vi "Check is Supported.vi"(10 "desired font(Application)":T2(ring), 11 "[user-specified font]":T1) -> (3 "is_supported":bool)   [LabVIEW 2021, in "Picture Pixel Fonts.lvlib"]
uses:
  <vilib>/LabVIEW Icon API/Pixel Fonts/Picture Pixel Fonts.lvlib
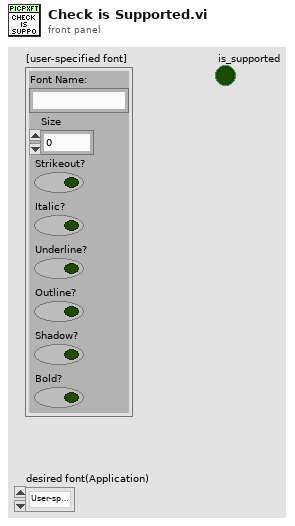
[diagram p1: front panel]
types:
  T1 = cluster{"Font Name:":string, "Size":i16, "Strikeout?":bool, "Italic?":bool, "Underline?":bool, "Outline?":bool, "Shadow?":bool, "Bold?":bool}
  T2 = enum16{"User-specified Font", "Application Font", "System Font", "Dialog Font"}
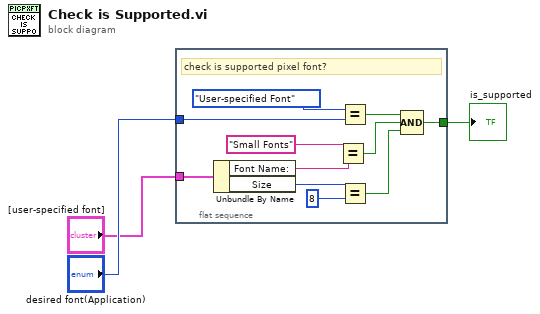
[diagram p0: block diagram]
diagram:
  n1 = flat-sequence {
    tunnel: "[user-specified font]" -> [w14]
    tunnel: "desired font(Application)" -> [w12]
    tunnel: [w4] -> w3
    frame #0 {
      # "check is supported pixel font?"
      n2 = Unbundle By Name(w14) -> ("Font Name:"=w11:string, "Size"=w7:i16)
      n3 = Equal?(x="Small Fonts" ("Font Name:"), y=w11) -> (x = y?=w9:bool)
      n4 = Equal?(x=T2."User-specified Font" ("desired font(Application)"), y=w12) -> (x = y?=w8:bool)
      n5 = Equal?(x=w7, y=i16 8) -> (x = y?=w5:bool)
      n6 = Compound Arithmetic op=AND(w8, w9, w5) -> (w4:bool)
    }
  }
  "is_supported" <- w3
